vi "Exemple_Metrics_Pairwise_Polynomial_Kernel.vi"() -> ()   [LabVIEW 2020]
uses:
  Objet/6 - Datasets Transformation/6.8 - Pairwise metrics, Affinities and Kernels/Polynomial_kernel/Polynomial_kernel.vi
panel:
  in  "polynomial_kernel":T1={"degree"=3, "gamma"="None", "coef0"=1.0}
  in  "error in":errorcluster caption="entrée d'erreur"
  in  "Y":string[][](array[string])=[["1", "0"], ["2", "1"]]
  in  "X":string[][](array[string])=[["2", "3"], ["3", "5"], ["5", "8"]]
  out "Data":T2
  out "error out":errorcluster caption="sortie d'erreur"
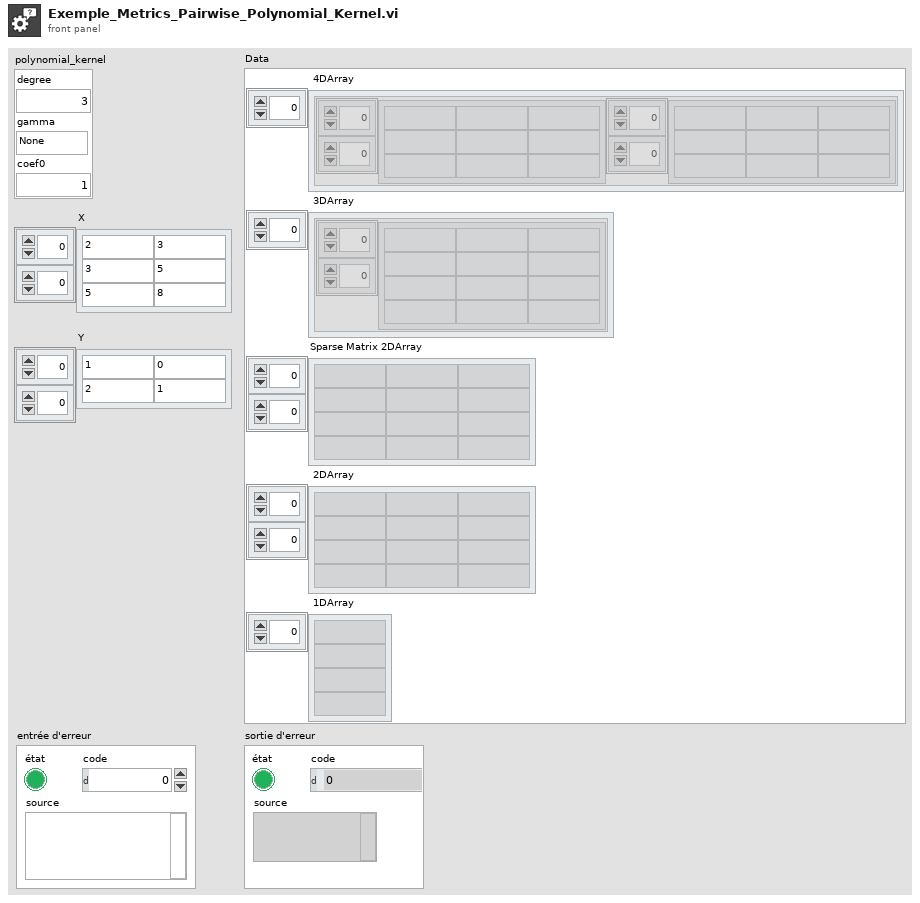
[diagram p1: front panel]
types:
  T1 = cluster{"degree":i32, "gamma":string, "coef0":dbl}
  T2 = cluster{" 4DArray":cluster{"1":string[][], "2":string[][]}[], " 3DArray":cluster{"Tableau":string[][]}[], "Sparse Matrix 2DArray":string[][], " 2DArray":string[][], " 1DArray":string[]}
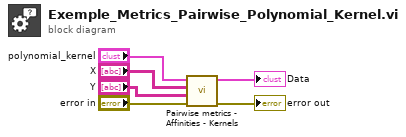
[diagram p0: block diagram]
diagram:
  n1 = call-poly "Pairwise metrics - Affinities - Kernels.vi"("error in"="error in", "Y"="Y", "X"="X", "polynomial_kernel"="polynomial_kernel") -> ("error out"=→"error out":errorcluster, "Data"=→"Data":T2)  [unwired: 6 in]
